vi "new XOR Filter.vi"(5 "a":refnum<class "Filter.lvclass">, 9 "b":refnum<class "Filter.lvclass">) -> (8 "a xor b":refnum<class "Filter.lvclass">)   [LabVIEW 2016, in "XOR Filter.lvclass"]
uses:
  XOR Filter.lvclass
  Filter Parent/Filter.lvclass
  C:/github/VeriStand-FPGA-Resource-Manager/Source/Client/Test CD/FPGA RM Test Client/Source/System Explorer/Filters/Filter Parent/Filter.lvclass
  XOR Filter.lvclass/XOR Filter.ctl
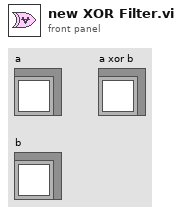
[diagram p1: front panel]
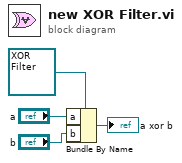
[diagram p0: block diagram]
diagram:
  n1 = Bundle By Name(cluster=refnum<class "XOR Filter.lvclass"> refnum ("XOR Filter in"), "a"="a", "b"="b") -> (→"a xor b":refnum<class "XOR Filter.lvclass">)
